vi "open Serial port.vi"(8 "error in (no error)":errorcluster caption="错误输入（无错误）", 11 "BD Protocol 4.0 输入":refnum<class "BD Protocol 4.0.lvclass">) -> (0 "error out":errorcluster caption="错误输出", 3 "BD Protocol 4.0 输出":refnum<class "BD Protocol 4.0.lvclass">)   [LabVIEW 2016, in "BD Protocol 4.0.lvlib" / "BD Protocol 4.0.lvclass"]
uses:
  BD Protocol 4.0.lvclass
  BD Protocol 4.0.lvclass/BD Protocol 4.0.ctl
  <vilib>/Instr/_visa.llb/VISA Configure Serial Port (Instr).vi
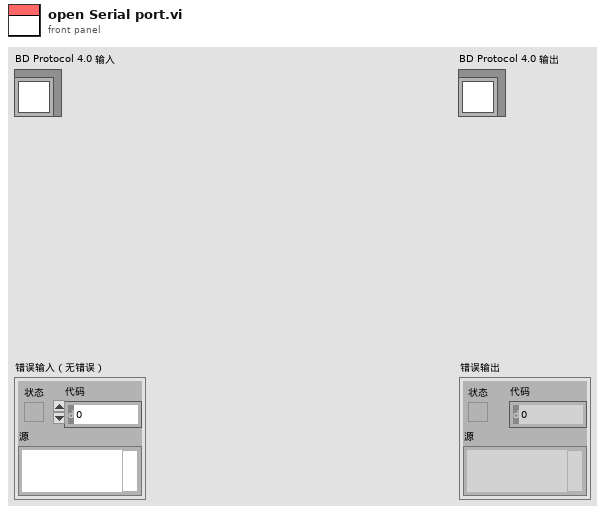
[diagram p1: front panel]
types:
  T1 = enum8{"Enabled", "Disabled", "Disabled and Grayed Out"}
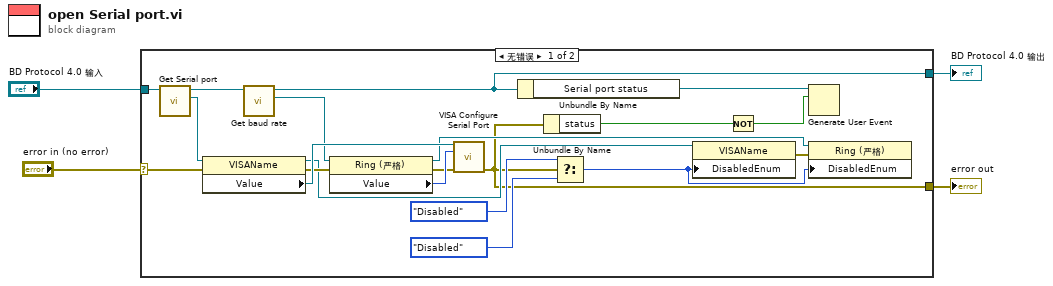
[diagram p0: block diagram]
diagram:
  n1 = case shown="无错误" "error in (no error)" {
    selector: "error in (no error)" -> [w12 w26]
    tunnel: [w5 w26] -> w3
    tunnel: [w13 w25] -> w1
    tunnel: "BD Protocol 4.0 输入" -> [w24 w25]
    frame No Error {
      n2 = call "Get Serial port.vi"("BD Protocol 4.0 in"=w24) -> ("Serial port"=w19:refnum<vi>, "BD Protocol 4.0 out"=w23:refnum<class "BD Protocol 4.0.lvclass">)  [unwired: 9 in]
      n3 = property class="VISAName"(reference=w19, error in=w12) -> (reference out=w10:refnum<vi>, error out=w16:errorcluster, "Value"=w18:refnum<visa-resource-name>)
      n4 = call "Get baud rate.vi"("BD Protocol 4.0 in"=w23) -> ("baud rate"=w17:refnum<vi>, "BD Protocol 4.0 out"=w13:refnum<class "BD Protocol 4.0.lvclass">)  [unwired: 9 in]
      n5 = property class="Ring (严格)"(reference=w17, error in=w16) -> (reference out=w9:refnum<vi>, error out=w14:errorcluster, "Value"=w15:u32)
      n6 = call-poly "VISA Configure Serial Port"("VISA resource name"=w18, "baud rate (9600)"=w15, "error in (no error)"=w14) -> ("error out"=w5:errorcluster)  [unwired: 11 in, 1 out]
      n7 = Unbundle By Name(w13) -> ("Serial port status"=w22:refnum<user-event>)
      n8 = Unbundle By Name(w5) -> ("status"=w21:bool)
      n9 = Select(t=T1."Disabled" ("禁用"), s=w5, f=T1."Disabled") -> (s? t:f=w6:T1)
      n10 = property class="VISAName"(reference=w10, "DisabledEnum"=w6) -> (error out=w11:errorcluster)  [unwired: 1 in, 1 out]
      n11 = Not(x=w21) -> (.not. x?=w20:bool)
      n12 = Generate User Event(user event=w22, event data cluster=w20) -> ()  [unwired: 2 in, 2 out]
      n13 = property class="Ring (严格)"(reference=w9, error in=w11, "DisabledEnum"=w6) -> ()  [unwired: 2 out]
    }
    frame Error {
    }
  }
  "error out" <- w3
  "BD Protocol 4.0 输出" <- w1
